vi "Actor Core.vi"(8 "error in":errorcluster, 11 "Example Sink in":refnum<class "Example Sink.lvclass">) -> (0 "error out":errorcluster, 3 "Actor out":refnum<class "Actor.lvclass">)   [LabVIEW 2016, in "Example Sink.lvlib" / "Example Sink.lvclass"]
doc: "(<B>Filename</B>: Actor Framework.lvlib:Actor.lvclass:Actor Core.vi)\n\nReceives messages to the actor, reacts to them, and initiates any error handling that may shut the actor down.\n\nDescendant classes may override this VI to append parallel tasks for the actor to complete while it handles messages. Overrides use the Call Parent Method node."
uses:
  Example Sink.lvclass
  <vilib>/ActorFramework/Actor/Actor.lvclass
  Example Sink.lvclass/Example Sink.ctl
  Event Sink/Event Sink.lvclass
panel:
  out "Time":string
  out "Waveform Graph":dbl[](graph)
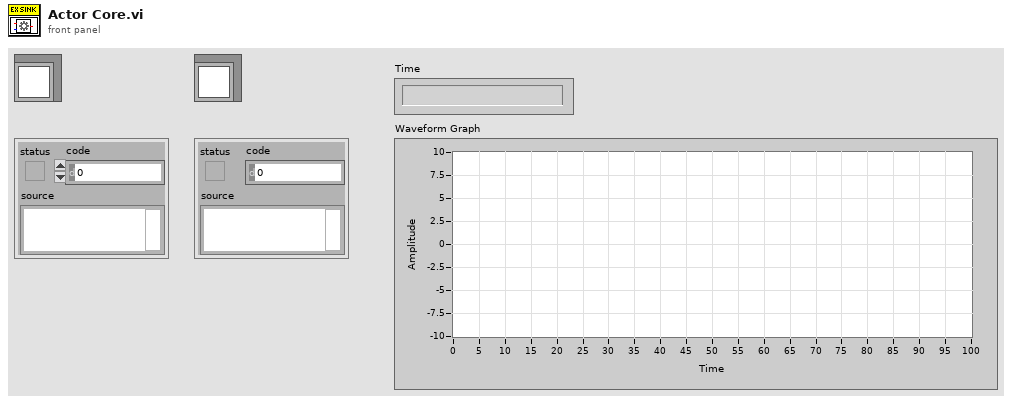
[diagram p1: front panel]
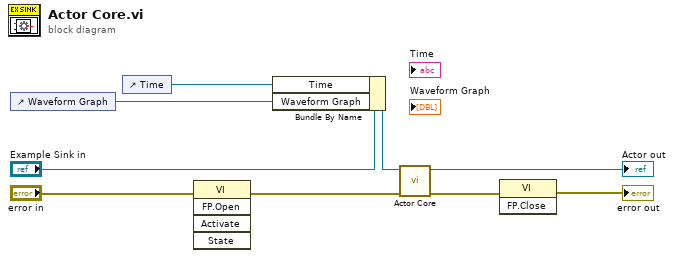
[diagram p0: block diagram]
diagram:
  n1 = control-ref of="Waveform Graph"() -> (w5:refnum<vi>)
  n2 = control-ref of="Time"() -> (w6:refnum<vi>)
  n3 = invoke class="VI" method="FP.Open"(error in="error in") -> (error out=w4:errorcluster)  [unwired: 4 in, 4 out]
  n4 = Bundle By Name(cluster="Example Sink in", "Time"=w6, "Waveform Graph"=w5) -> (w7:refnum<class "Example Sink.lvclass">)
  n5 = call-parent "Actor Core.vi"("error in"=w4, "Actor in"=w7) -> ("error out"=w3:errorcluster, "Actor out"=→"Actor out":refnum<class "Actor.lvclass">)  [unwired: 8 in]
  n6 = invoke class="VI" method="FP.Close"(error in=w3) -> (error out=→"error out":errorcluster)  [unwired: 2 in, 2 out]
